vi "Periodic Tasks_Hue.vi"(8 "error in":errorcluster, 11 "RobotConfig":T7={"Motors"={"RightDrivePrimary"={"CAN Address"=0, "Invert"=FALSE, "InvertSensor"=FALSE, "Unit Conversion Factor"=0.0, "Brake Mode"=enum."Override to Brake", "Reverse Limt Switch Mode"=enum."Disabled", "Forward Limt Swith Mode"=enum."Disabled", "PWM Channel"=enum."Invalid", "Motor Controller Type"=enum."Talon SRX", "Peak Current (A)"=0, "Continuous Current (A)"=0, "Peak Duration (ms)"=0, "Current Limit Enable"=FALSE}, "RightDriveSecondary"={"CAN Address"=0, "Invert"=FALSE, "InvertSensor"=FALSE, "Unit Conversion Factor"=0.0, "Brake Mode"=enum."Override to Brake", "Reverse Limt Switch Mode"=enum."Disabled", "Forward Limt Swith Mode"=enum."Disabled", "PWM Channel"=enum."Invalid", "Motor Controller Type"=enum."Talon SRX", "Peak Current (A)"=0, "Continuous Current (A)"=0, "Peak Duration (ms)"=0, "Current Limit Enable"=FALSE}, "LeftDrivePrimary"={"CAN Address"=0, "Invert"=FALSE, "InvertSensor"=FALSE, "Unit Conversion Factor"=0.0, "Brake Mode"=enum."Override to Brake", "Reverse Limt Switch Mode"=enum."Disabled", "Forward Limt Swith Mode"=enum."Disabled", "PWM Channel"=enum."Invalid", "Motor Controller Type"=enum."Talon SRX", "Peak Current (A)"=0, "Continuous Current (A)"=0, "Peak Duration (ms)"=0, "Current Limit Enable"=FALSE}, "LeftDriveSecondary"={"CAN Address"=0, "Invert"=FALSE, "InvertSensor"=FALSE, "Unit Conversion Factor"=0.0, "Brake Mode"=enum."Override to Brake", "Reverse Limt Switch Mode"=enum."Disabled", "Forward Limt Swith Mode"=enum."Disabled", "PWM Channel"=enum."Invalid", "Motor Controller Type"=enum."Talon SRX", "Peak Current (A)"=0, "Continuous Current (A)"=0, "Peak Duration (ms)"=0, "Current Limit Enable"=FALSE}, "RightShooter"={"CAN Address"=0, "Invert"=FALSE, "InvertSensor"=FALSE, "Unit Conversion Factor"=0.0, "Brake Mode"=enum."Override to Brake", "Reverse Limt Switch Mode"=enum."Disabled", "Forward Limt Swith Mode"=enum."Disabled", "PWM Channel"=enum."Invalid", "Motor Controller Type"=enum."Talon SRX", "Peak Current (A)"=0, "Continuous Current (A)"=0, "Peak Duration (ms)"=0, "Current Limit Enable"=FALSE}, "LeftShooter"={"CAN Address"=0, "Invert"=FALSE, "InvertSensor"=FALSE, "Unit Conversion Factor"=0.0, "Brake Mode"=enum."Override to Brake", "Reverse Limt Switch Mode"=enum."Disabled", "Forward Limt Swith Mode"=enum."Disabled", "PWM Channel"=enum."Invalid", "Motor Controller Type"=enum."Talon SRX", "Peak Current (A)"=0, "Continuous Current (A)"=0, "Peak Duration (ms)"=0, "Current Limit Enable"=FALSE}, "ShooterRotate"={"CAN Address"=0, "Invert"=FALSE, "InvertSensor"=FALSE, "Unit Conversion Factor"=0.0, "Brake Mode"=enum."Override to Brake", "Reverse Limt Switch Mode"=enum."Disabled", "Forward Limt Swith Mode"=enum."Disabled", "PWM Channel"=enum."Invalid", "Motor Controller Type"=enum."Talon SRX", "Peak Current (A)"=0, "Continuous Current (A)"=0, "Peak Duration (ms)"=0, "Current Limit Enable"=FALSE}, "ShooterHood"={"CAN Address"=0, "Invert"=FALSE, "InvertSensor"=FALSE, "Unit Conversion Factor"=0.0, "Brake Mode"=enum."Override to Brake", "Reverse Limt Switch Mode"=enum."Disabled", "Forward Limt Swith Mode"=enum."Disabled", "PWM Channel"=enum."Invalid", "Motor Controller Type"=enum."Talon SRX", "Peak Current (A)"=0, "Continuous Current (A)"=0, "Peak Duration (ms)"=0, "Current Limit Enable"=FALSE}, "HopperWheel"={"CAN Address"=0, "Invert"=FALSE, "InvertSensor"=FALSE, "Unit Conversion Factor"=0.0, "Brake Mode"=enum."Override to Brake", "Reverse Limt Switch Mode"=enum."Disabled", "Forward Limt Swith Mode"=enum."Disabled", "PWM Channel"=enum."Invalid", "Motor Controller Type"=enum."Talon SRX", "Peak Current (A)"=0, "Continuous Current (A)"=0, "Peak Duration (ms)"=0, "Current Limit Enable"=FALSE}, "Elevator"={"CAN Address"=0, "Invert"=FALSE, "InvertSensor"=FALSE, "Unit Conversion Factor"=0.0, "Brake Mode"=enum."Override to Brake", "Reverse Limt Switch Mode"=enum."Disabled", "Forward Limt Swith Mode"=enum."Disabled", "PWM Channel"=enum."Invalid", "Motor Controller Type"=enum."Talon SRX", "Peak Current (A)"=0, "Continuous Current (A)"=0, "Peak Duration (ms)"=0, "Current Limit Enable"=FALSE}, "ClimberLeft"={"CAN Address"=0, "Invert"=FALSE, "InvertSensor"=FALSE, "Unit Conversion Factor"=0.0, "Brake Mode"=enum."Override to Brake", "Reverse Limt Switch Mode"=enum."Disabled", "Forward Limt Swith Mode"=enum."Disabled", "PWM Channel"=enum."Invalid", "Motor Controller Type"=enum."Talon SRX", "Peak Current (A)"=0, "Continuous Current (A)"=0, "Peak Duration (ms)"=0, "Current Limit Enable"=FALSE}, "ClimberRight"={"CAN Address"=0, "Invert"=FALSE, "InvertSensor"=FALSE, "Unit Conversion Factor"=0.0, "Brake Mode"=enum."Override to Brake", "Reverse Limt Switch Mode"=enum."Disabled", "Forward Limt Swith Mode"=enum."Disabled", "PWM Channel"=enum."Invalid", "Motor Controller Type"=enum."Talon SRX", "Peak Current (A)"=0, "Continuous Current (A)"=0, "Peak Duration (ms)"=0, "Current Limit Enable"=FALSE}, "Intake"={"CAN Address"=0, "Invert"=FALSE, "InvertSensor"=FALSE, "Unit Conversion Factor"=0.0, "Brake Mode"=enum."Override to Brake", "Reverse Limt Switch Mode"=enum."Disabled", "Forward Limt Swith Mode"=enum."Disabled", "PWM Channel"=enum."Invalid", "Motor Controller Type"=enum."Talon SRX", "Peak Current (A)"=0, "Continuous Current (A)"=0, "Peak Duration (ms)"=0, "Current Limit Enable"=FALSE}, "ControlPanel"={"CAN Address"=0, "Invert"=FALSE, "InvertSensor"=FALSE, "Unit Conversion Factor"=0.0, "Brake Mode"=enum."Override to Brake", "Reverse Limt Switch Mode"=enum."Disabled", "Forward Limt Swith Mode"=enum."Disabled", "PWM Channel"=enum."Invalid", "Motor Controller Type"=enum."Talon SRX", "Peak Current (A)"=0, "Continuous Current (A)"=0, "Peak Duration (ms)"=0, "Current Limit Enable"=FALSE}}, "PID"={"Shooter"={"P"=0.0, "I"=0.0, "D"=0.0, "F"=0.0, "IZone"=0.0}, "Turret"={"P"=0.0, "I"=0.0, "D"=0.0, "F"=0.0, "IZone"=0.0}, "Elevator"={"P"=0.0, "I"=0.0, "D"=0.0, "F"=0.0, "IZone"=0.0}, "ControlPanel"={"P"=0.0, "I"=0.0, "D"=0.0, "F"=0.0, "IZone"=0.0}, "Hood"={"P"=0.0, "I"=0.0, "D"=0.0, "F"=0.0, "IZone"=0.0}}, "MotionMagic"={"Turret"={"CruiseVelocity"=0, "Acceleration"=0}, "Elevator"={"CruiseVelocity"=0, "Acceleration"=0}, "ControlPanel"={"CruiseVelocity"=0, "Acceleration"=0}}, "Sensors"={"IMU"={"Yaw Axis"=enum."Z", "SPI Bus"=enum."SPI MXP", "AHRS Algorithm"=enum."Complementary", "Calibration Time (s)"=3.0, "Calibrate On Open"=TRUE}, "ElevatorBottom"={"ID"=0, "RangingMode"=enum."Short", "sampleTime(ms)"=24.0}, "ElevatorTop"={"ID"=0, "RangingMode"=enum."Short", "sampleTime(ms)"=24.0}}, "Solenoids"={"Intake"={"SolenoidChannel"=enum."Solenoid 0", "Invert"=FALSE}, "ClimberRachet"={"SolenoidChannel"=enum."Solenoid 0", "Invert"=FALSE}}, "EnableCompressor"=FALSE, "RobotDimensions"={"Wheelbase(in)"=0.0, "Length(in)"=0.0}, "CameraMounting"={"LensHeight(in)"=0.0, "RotationRadius(in)"=0.0, "Pitch(deg)"=0.0}, "SensorCalibrations"={"TopToFMinBallDistance(in)"=0.0, "BottomToFMinBallDistance(in)"=0.0}, "Homing"={"Hood Homing Position (deg)"=0.0, "Turret Homing Position (deg)"=0.0}, "MotionLimits"={"Hood"={"Min (deg)"=0.0, "Max (deg)"=0.0}, "Turret"={"Min (deg)"=0.0, "Max (deg)"=0.0}}} {"Sensors"."ElevatorTop"."sampleTime(ms)" min=24.0 max=1000.0 step=1.0; "Sensors"."ElevatorBottom"."sampleTime(ms)" min=24.0 max=1000.0 step=1.0}) -> ()   [LabVIEW 2019]
doc: "This VI runs in parallel to other tasks. It can contain as many user-defined periodic loops as you need. These can carry out PID or other sorts of timed response."
uses:
  InfiniteRechargeSrc/TypeDefs/ConfigComponents/Config_Robot.ctl
  ArgosLib/Config/ConfigComponents/TypeDefs/Config_Motor.ctl
  <vilib>/Rock Robotics/WPI/ThirdParty/Phoenix-LabVIEW/Motor Controller/Controls/CTRE_Phoenix_MotorControl_NeutralMode.ctl
  <vilib>/Rock Robotics/WPI/ThirdParty/Phoenix-LabVIEW/Motor Controller/Controls/CTRE_Phoenix_MotorControl_LimitSwitchNormal.ctl
  <vilib>/Rock Robotics/SystemInterfaces/DIO/FPGA_DIOPWMChannel.ctl
  ArgosLib/Config/ConfigComponents/TypeDefs/Config_MotorCtrlType.ctl
  ArgosLib/Config/ConfigComponents/TypeDefs/Config_PIDParams.ctl
  ArgosLib/Config/ConfigComponents/TypeDefs/Config_MotionMagicParams.ctl
  ArgosLib/Config/ConfigComponents/TypeDefs/Config_IMU.ctl
  <vilib>/Rock Robotics/SystemInterfaces/spilib/spi_bus.ctl
  ArgosLib/Config/ConfigComponents/TypeDefs/Config_PwFToF.ctl
  <vilib>/Playing With Fusion Inc/Playing With Fusion Lib for FRC/PWF_ToF_LabVIEW/Public/TypeDefs/PwF_ToF_RangingMode.ctl
  ArgosLib/Config/ConfigComponents/TypeDefs/Config_SingleSolenoid.ctl
  <vilib>/Rock Robotics/WPI/Solenoid/WPI_SolenoidChannel.ctl
  InfiniteRechargeSrc/TypeDefs/ConfigComponents/Config_RobotDimensions.ctl
  InfiniteRechargeSrc/TypeDefs/ConfigComponents/Config_CameraMounting.ctl
  ArgosLib/Miscellaneous/TypeDefs/ArgoDriveJoystickMap.ctl
  ArgosLib/Miscellaneous/TypeDefs/LookUpTableParameters.ctl
  InfiniteRechargeSrc/Implements/Shooter/TypeDefs/Hood_Homing_State.ctl
  <vilib>/Playing With Fusion Inc/Playing With Fusion Lib for FRC/PWF_TMD37003_LabVIEW/Public/TypeDefs/PwF_TMD37003_Data.ctl
  <vilib>/Playing With Fusion Inc/Playing With Fusion Lib for FRC/PWF_TMD37003_LabVIEW/Public/TypeDefs/PwF_TMD37003_Gains.ctl
  InfiniteRechargeSrc/Implements/Control_Panel/TypeDefs/ControlPanelColor.ctl
  InfiniteRechargeSrc/Vision/TypeDefs/VisionPipeline.ctl
  <vilib>/Rock Robotics/WPI/Utilities/WPI_GetSetVariantRefNum.vi
  InfiniteRechargeSrc/Global_Var-RefNum/JoystickControls.vi
  <vilib>/Playing With Fusion Inc/Playing With Fusion Lib for FRC/PWF_TMD37003_LabVIEW/Public/PwF_TMD37003_RGBToHSV_SensorData.vi
  ArgosLib/ArgosLib.lvlib
  <vilib>/Playing With Fusion Inc/Playing With Fusion Lib for FRC/PWF_TMD37003_LabVIEW/PwF_TMD37003.lvlib
  <vilib>/Playing With Fusion Inc/Playing With Fusion Lib for FRC/PWF_ToF_LabVIEW/PwF_ToF.lvlib
panel:
  out "Color":T1
  out "Hue":dbl
  in  "TMD37003Gains":T2={"rGain"=5.0761, "gGain"=7.9365, "bGain"=14.0845, "cGain"=2.9411, "gamma"=0.4545}
  in  "alsGain":u8=40
  in  "alsIntegrationTime(ms)":dbl=10.0
  out "TMD37003 Data":T3
  in  "ShooterSpeed(rpm)":dbl(slide)=4000.0 min=0.0 max=7000.0 step=1.0 scale=0.0..7000.0
  in  "DisableLimelight":bool
  out "Target Found?":bool
  in  "SetPointTurret(Deg)":dbl(slide) scale=-108.0..108.0
  in  "Activate Auto (Turret)":bool
  out "TurretManual":bool
  out "Turret Current Position (Deg)":dbl
  out "Hood Current Position (Deg)":dbl
  out "HoodManual?":bool
  in  "Activate Auto (Shooter Hood)":bool
  in  "SetPointHood(Deg)":dbl
  in  "TurretHomeReset":bool
  in  "Turret Homing Activated":bool
  out "Turret Homing_State":T4
  in  "HoodHomeActivate":bool
  in  "HoodHomeReset":bool
  out "Hood_Homing_State":T4
  in  "Argo Drive Joystick Map":T5={"Auto Speed"={"Look Up Table OUT"=[-1.0, 0.0, 1.0], "Look Up Table IN"=[-1.0, 0.0, 1.0]}, "Low Speed"={"Look Up Table OUT"=[-1.0, 0.0, 0.0, 1.0], "Look Up Table IN"=[-1.0, -0.25, 0.25, 1.0]}, "Auto Turning"={"Look Up Table OUT"=[-1.0, 0.0, 1.0], "Look Up Table IN"=[-1.0, 0.0, 1.0]}, "Low Turning"={"Look Up Table OUT"=[-1.0, 0.0, 0.0, 1.0], "Look Up Table IN"=[-1.0, -0.25, 0.25, 1.0]}, "High Speed"={"Look Up Table OUT"=[], "Look Up Table IN"=[]}, "High Turning"={"Look Up Table OUT"=[], "Look Up Table IN"=[]}}
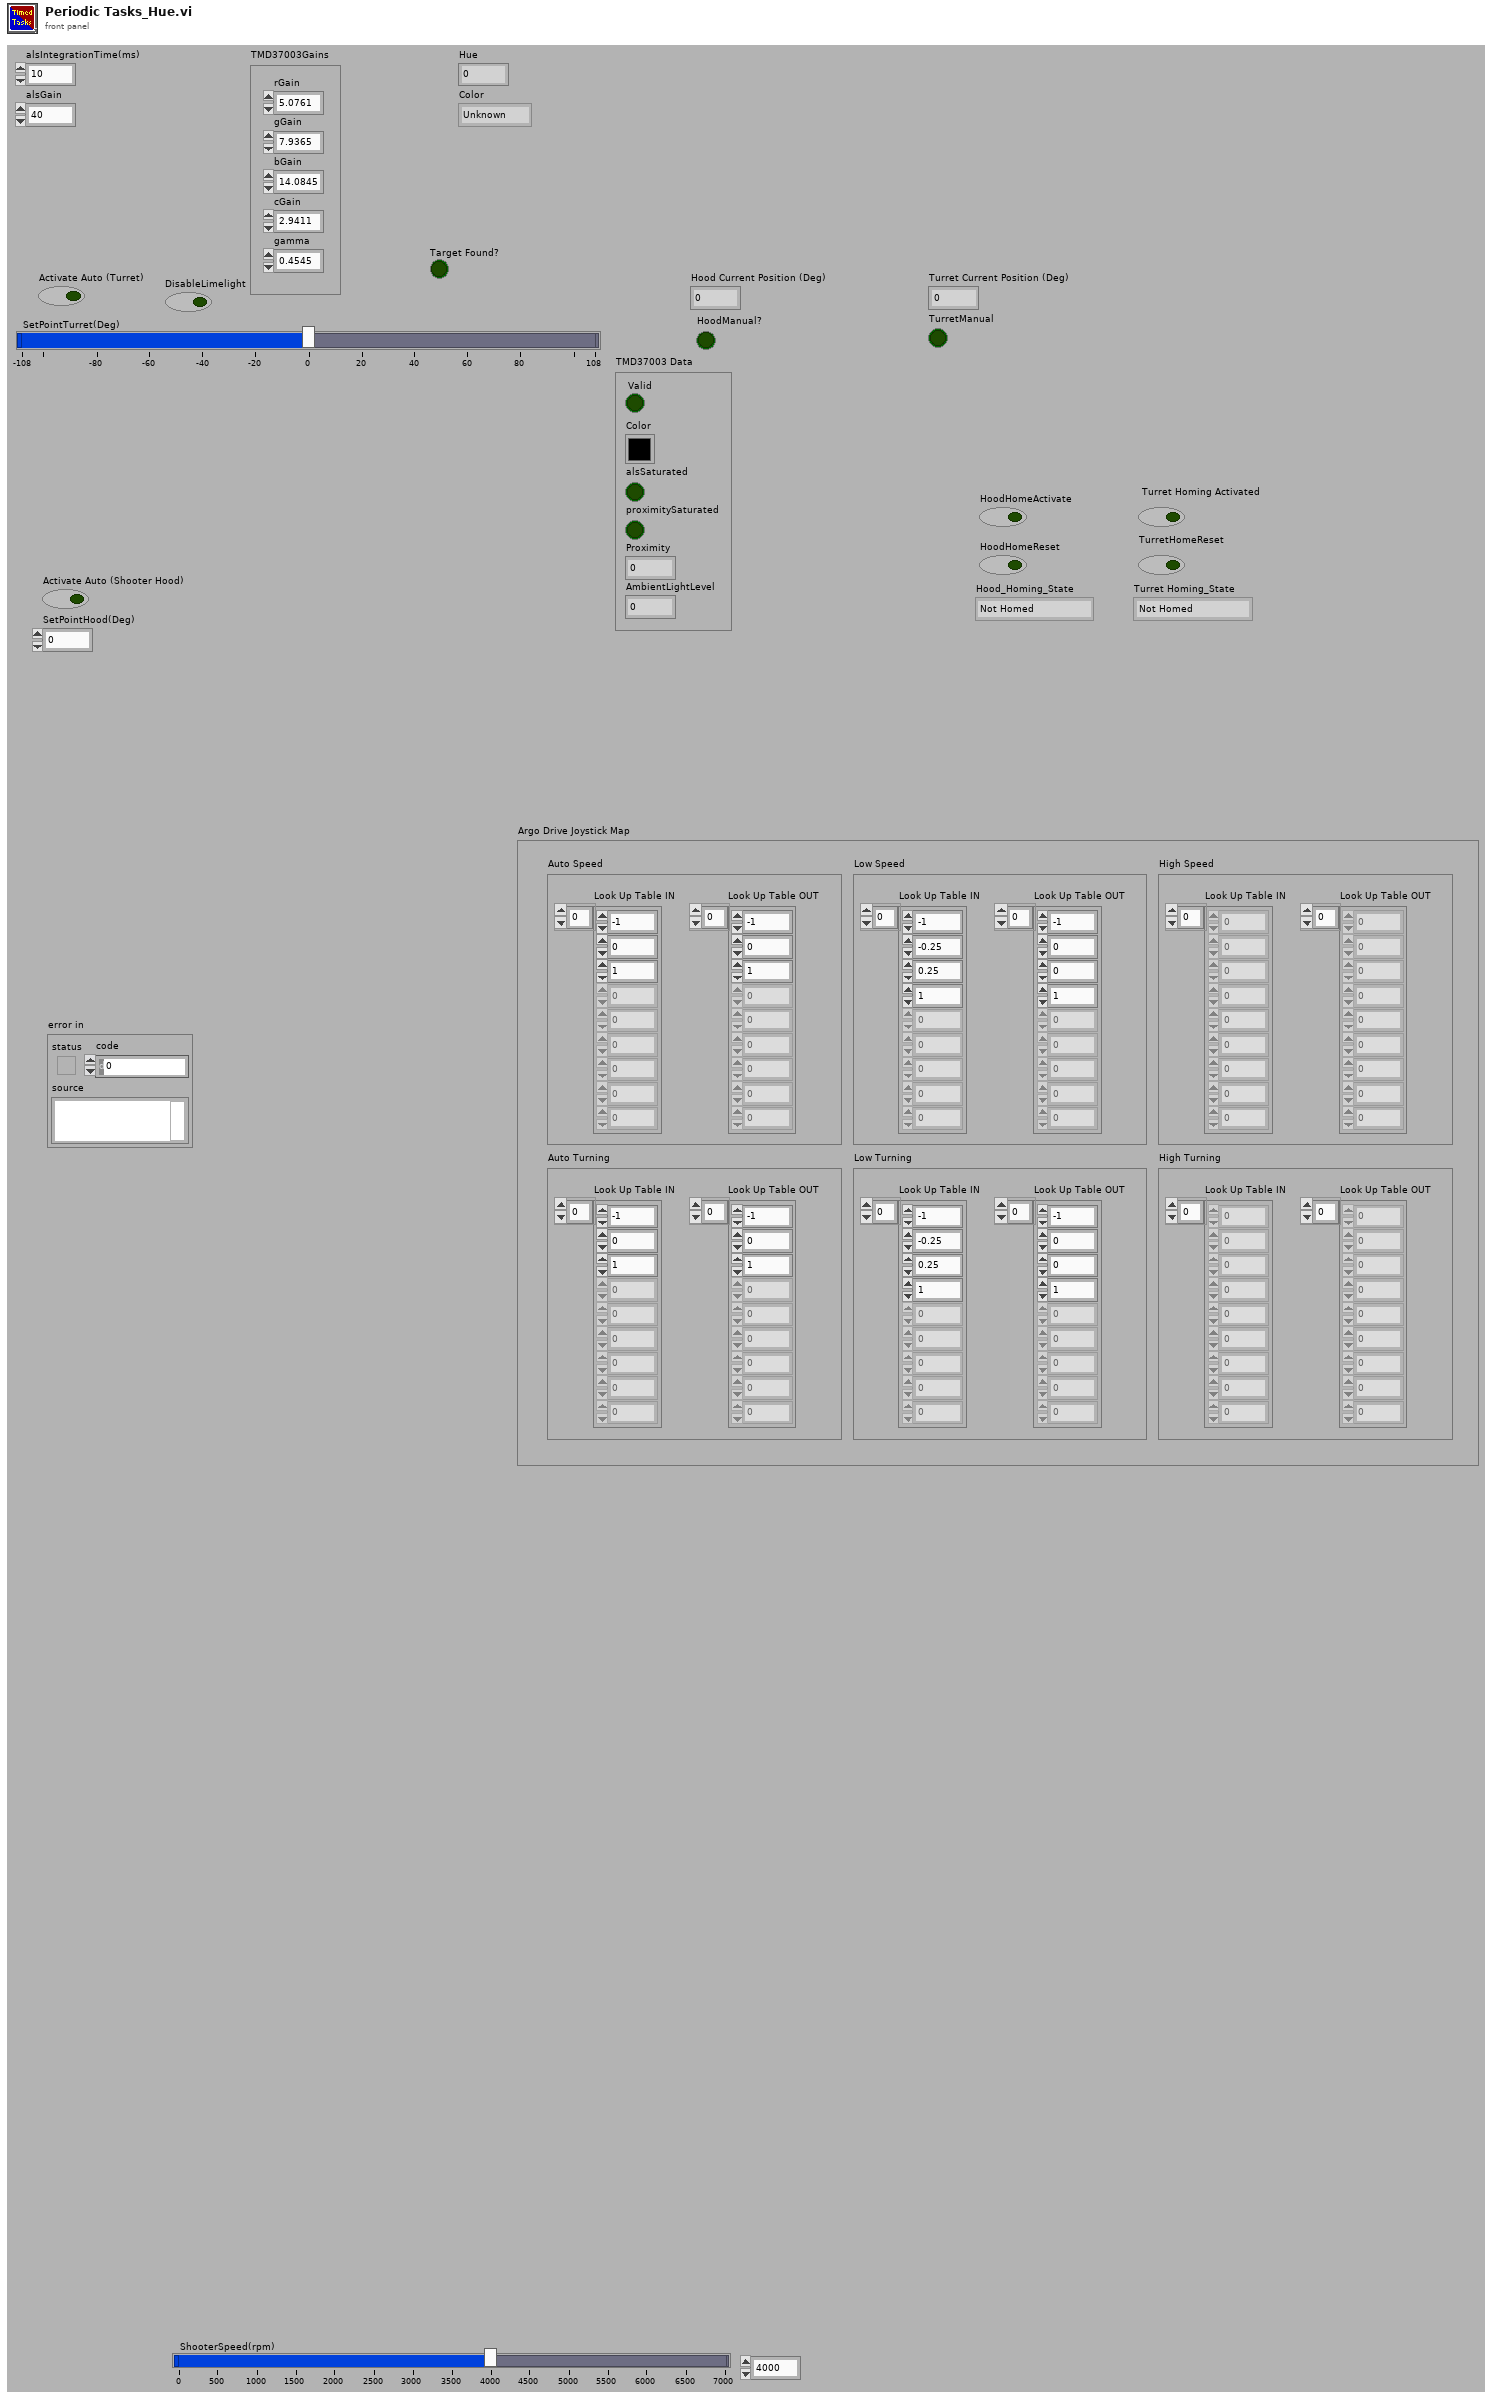
[diagram p1: front panel]
types:
  T1 = typedef "ControlPanelColor.ctl" = enum16{"Unknown", "Red", "Green", "Blue", "Yellow"}
  T2 = typedef "PlayingWithFusionLib.lvlib/PwF_TMD37003.lvlib/PwF_TMD37003_Gains.ctl" = cluster{"rGain":dbl, "gGain":dbl, "bGain":dbl, "cGain":dbl, "gamma":dbl}
  T3 = typedef "PlayingWithFusionLib.lvlib/PwF_TMD37003.lvlib/PwF_TMD37003_Data.ctl" = cluster{"Valid":bool, "Color":u32, "alsSaturated":bool, "proximitySaturated":bool, "Proximity":dbl, "AmbientLightLevel":dbl}
  T4 = typedef "Hood_Homing_State.ctl" = enum16{"Not Homed", "Homing in Process", "Homing Failed", "Homing Completed"}
  T5 = typedef "ArgosLib.lvlib/ArgoDriveJoystickMap.ctl" = cluster{"Auto Speed":T6, "Low Speed":T6, "Auto Turning":T6, "Low Turning":T6, "High Speed":T6, "High Turning":T6}
  T6 = typedef "ArgosLib.lvlib/LookUpTableParameters.ctl" = cluster{"Look Up Table OUT":dbl[], "Look Up Table IN":dbl[]}
  T7 = typedef "Config_Robot.ctl" = cluster{"Motors":cluster{"RightDrivePrimary":T8, "RightDriveSecondary":T8, "LeftDrivePrimary":T8, "LeftDriveSecondary":T8, "RightShooter":T8, "LeftShooter":T8, "ShooterRotate":T8, "ShooterHood":T8, "HopperWheel":T8, "Elevator":T8, "ClimberLeft":T8, "ClimberRight":T8, "Intake":T8, "ControlPanel":T8}, "PID":cluster{"Shooter":T13, "Turret":T13, "Elevator":T13, "ControlPanel":T13, "Hood":T13}, "MotionMagic":cluster{"Turret":T14, "Elevator":T14, "ControlPanel":T14}, "Sensors":cluster{"IMU":T15, "ElevatorBottom":T17, "ElevatorTop":T17}, "Solenoids":cluster{"Intake":T19, "ClimberRachet":T19}, "EnableCompressor":bool, "RobotDimensions":T21, "CameraMounting":T22, "SensorCalibrations":cluster{"TopToFMinBallDistance(in)":dbl, "BottomToFMinBallDistance(in)":dbl}, "Homing":cluster{"Hood Homing Position (deg)":dbl, "Turret Homing Position (deg)":dbl}, "MotionLimits":cluster{"Hood":cluster{"Min (deg)":dbl, "Max (deg)":dbl}, "Turret":cluster{"Min (deg)":dbl, "Max (deg)":dbl}}}
  T8 = typedef "ArgosLib.lvlib/Config_Motor.ctl" = cluster{"CAN Address":u8, "Invert":bool, "InvertSensor":bool, "Unit Conversion Factor":dbl, "Brake Mode":T9, "Reverse Limt Switch Mode":T10, "Forward Limt Swith Mode":T10, "PWM Channel":T11, "Motor Controller Type":T12, "Peak Current (A)":i32, "Continuous Current (A)":i32, "Peak Duration (ms)":i32, "Current Limit Enable":bool}
  T9 = typedef "CTRE_Phoenix_MotorControl_NeutralMode.ctl" = enum8{"EEPROMSetting", "Override to Coast", "Override to Brake"}
  T10 = typedef "CTRE_Phoenix_MotorControl_LimitSwitchNormal.ctl" = enum16{"Normally Open", "Normally Closed", "Disabled"}
  T11 = typedef "FPGA_DIOPWMChannel.ctl" = enum8{"PWM 0", "PWM 1", "PWM 2", "PWM 3", "PWM 4", "PWM 5", "PWM 6", "PWM 7", "PWM 8", "PWM 9", "PWM MXP 0", "PWM MXP 1", "PWM MXP 2", "PWM MXP 3", "PWM MXP 4", "PWM MXP 5", "PWM MXP 6", "PWM MXP 7", "PWM MXP 8", "PWM MXP 9", "Invalid"}
  T12 = typedef "ArgosLib.lvlib/Config_MotorCtrlType.ctl" = enum16{"Disabled", "Talon SRX", "Talon SR", "Venom", "Spark MAX"}
  T13 = typedef "ArgosLib.lvlib/Config_PIDParams.ctl" = cluster{"P":dbl, "I":dbl, "D":dbl, "F":dbl, "IZone":dbl}
  T14 = typedef "ArgosLib.lvlib/Config_MotionMagicParams.ctl" = cluster{"CruiseVelocity":i32, "Acceleration":i32}
  T15 = typedef "ArgosLib.lvlib/Config_IMU.ctl" = cluster{"Yaw Axis":enum16{"X", "Y", "Z"}, "SPI Bus":T16, "AHRS Algorithm":enum16{"Complementary", "Madgwick"}, "Calibration Time (s)":dbl, "Calibrate On Open":bool}
  T16 = typedef "spi_bus.ctl" = enum16{"SPI On-Board, CS0", "SPI On-Board, CS1", "SPI On-Board, CS2", "SPI On-Board, CS3", "SPI MXP", "Invalid"}
  T17 = typedef "ArgosLib.lvlib/Config_PwFToF.ctl" = cluster{"ID":u8, "RangingMode":T18, "sampleTime(ms)":dbl}
  T18 = typedef "PlayingWithFusionLib.lvlib/PwF_ToF.lvlib/PwF_ToF_RangingMode.ctl" = enum16{"Short", "Medium", "Long"}
  T19 = typedef "ArgosLib.lvlib/Config_SingleSolenoid.ctl" = cluster{"SolenoidChannel":T20, "Invert":bool}
  T20 = typedef "WPI_SolenoidChannel.ctl" = enum8{"Solenoid 0", "Solenoid 1", "Solenoid 2", "Solenoid 3", "Solenoid 4", "Solenoid 5", "Solenoid 6", "Solenoid 7", "Invalid"}
  T21 = typedef "Config_RobotDimensions.ctl" = cluster{"Wheelbase(in)":dbl, "Length(in)":dbl}
  T22 = typedef "Config_CameraMounting.ctl" = cluster{"LensHeight(in)":dbl, "RotationRadius(in)":dbl, "Pitch(deg)":dbl}
  T23 = typedef "SensorRefNums.ctl" = cluster{"ElevatorBottom":T24, "ElevatorTop":T24}
  T24 = typedef "PlayingWithFusionLib.lvlib/PwF_ToF.lvlib/PwF_ToF_DevRef.ctl" = cluster{"DeviceStatus":errorcluster, "Device Number":u8, "Handle":u64, "Library Path":path}
  T25 = typedef "JoystickRefNums.ctl" = cluster{"Joystick0":T26, "Joystick1":T26}
  T26 = typedef "WPI_JoystickDevRef.ctl" = cluster{"Device":T27}
  T27 = typedef "WPI_JoystickDeviceEnum.ctl" = enum16{"USB 0", "USB 1", "USB 2", "USB 3", "USB 4", "USB 5"}
  T28 = typedef "WPI_RobotDriveDevRef.ctl" = cluster{"DevStatus":errorcluster, "Motors[]":T29[], "Square Inputs":bool, "Max Output":dbl}
  T29 = typedef "WPI_MotorControlDeviceRef.ctl" = cluster{"DeviceStatus":errorcluster, "Type":T30, "PWM":cluster{"PWM Channel":T11, "DeadBand":T31}, "CAN":cluster{"Device Number":u8, "SetOutput VI Ref":variant, "GetOutput VI Ref":variant, "Enable VI Ref":variant, "Disable VI Ref":variant, "Data":variant}, "Invert":bool, "DIO PWM":cluster{"PWM \"Enable\" Channel":T11, "DIOChannel":T32, "PWM Rate":dbl}}
  T30 = typedef "WPI_MotorControlType.ctl" = enum16{"PWM", "CAN", "DIO PWM"}
  T31 = typedef "WPI_PWMDeadband.ctl" = cluster{"Name":string, "maxPositivePwm":i32, "minPositivePwm":i32, "centerPwm":i32, "maxNegativePwm":i32, "minNegativePwm":i32, "angularRange":u16}
  T32 = typedef "FPGA_DIOChannel.ctl" = enum8{"DIO 0", "DIO 1", "DIO 2", "DIO 3", "DIO 4", "DIO 5", "DIO 6", "DIO 7", "DIO 8", "DIO 9", "DIO MXP 0", "DIO MXP 1", "DIO MXP 2", "DIO MXP 3", "DIO MXP 4", "DIO MXP 5", "DIO MXP 6", "DIO MXP 7", "DIO MXP 8", "DIO MXP 9", "DIO MXP 10", "DIO MXP 11", "DIO MXP 12", "DIO MXP 13", "DIO MXP 14", "DIO MXP 15", "SPI Port CS1", "SPI Port CS2", "SPI Port CS3", "SPI Port MISO", "SPI Port MOSI", "Invalid"}
  T33 = typedef "PneumaticsRefNums.ctl" = cluster{"Intake":T34, "Compressor":T35, "ClimberRatchet":T34}
  T34 = typedef "WPI_SolenoidDevRef.ctl" = cluster{"DevStatus":errorcluster, "Pneumatics Control Module":u8, "Forward Solenoid Channel":T20, "Reverse Solenoid Channel":T20}
  T35 = typedef "WPI_CompressorDevRef.ctl" = cluster{"DevStatus":errorcluster, "Pneumatics Control Module":u8}
  T36 = typedef "MotorRefNums.ctl" = cluster{"LeftDrivePrimary":T29, "RightDrivePrimary":T29, "LeftDriveSecondary":T29, "RightDriveSecondary":T29, "RightShooter":T29, "LeftShooter":T29, "ShooterRotate":T29, "ShooterHood":T29, "HopperWheel":T29, "Elevator":T29, "ClimberLeft":T29, "ClimberRight":T29, "Intake":T29, "ControlPanel":T29}
  T37 = cluster{"RobotConfig":T7, "JoystickRefNums":T25, "RobotDriveDevRef":T28, "MotorRefNumsOut":T36, "Pneumatics":T33, "Sensors":T23}
  T38 = typedef "PlayingWithFusionLib.lvlib/PwF_TMD37003.lvlib/PwF_TMD37003_DevRef.ctl" = cluster{"DevStatus":errorcluster, "Device Address":u8, "Handle":i32, "I2C Bus":T39}
  T39 = typedef "i2c_bus.ctl" = enum16{"I2C On-Board", "I2C MXP", "Invalid"}
  T40 = typedef "JoystickControl.ctl" = cluster{"A":bool, "B":bool, "X":bool, "Y":bool, "LB":bool, "Shoot":bool, "LJ":bool, "RJ":bool, "Back":bool, "Start":bool, "Top":bool, "Right":bool, "Bottom":bool, "Left":bool, "Eject":dbl, "Intake":dbl, "LX":dbl, "Drive Y":dbl, "Drive X":dbl, "RY":dbl, "Down":bool, "Index":bool, "Aggitate":bool, "Up":bool, "Find Target":bool, "Spin up":bool, "LJ 2":bool, "RJ 2":bool, "Back 2":bool, "Start 2":bool, "Elevate":bool, "Right 2":bool, "Retract":bool, "Left 2":bool, "Control Rotate":dbl, "RT 2":dbl, "H L/R":dbl, "H U/D":dbl, "RX 2":dbl, "RY 2":dbl}
  T41 = typedef "VisionPipeline.ctl" = enum16{"LEDOff", "NoZoom", "Zoom2x", "Zoom3x"}
  T42 = typedef "VisionTarget.ctl" = cluster{"Valid":bool, "Distance(in)":dbl, "Angle(deg)":dbl, "FieldCentricAngle(deg)":dbl}
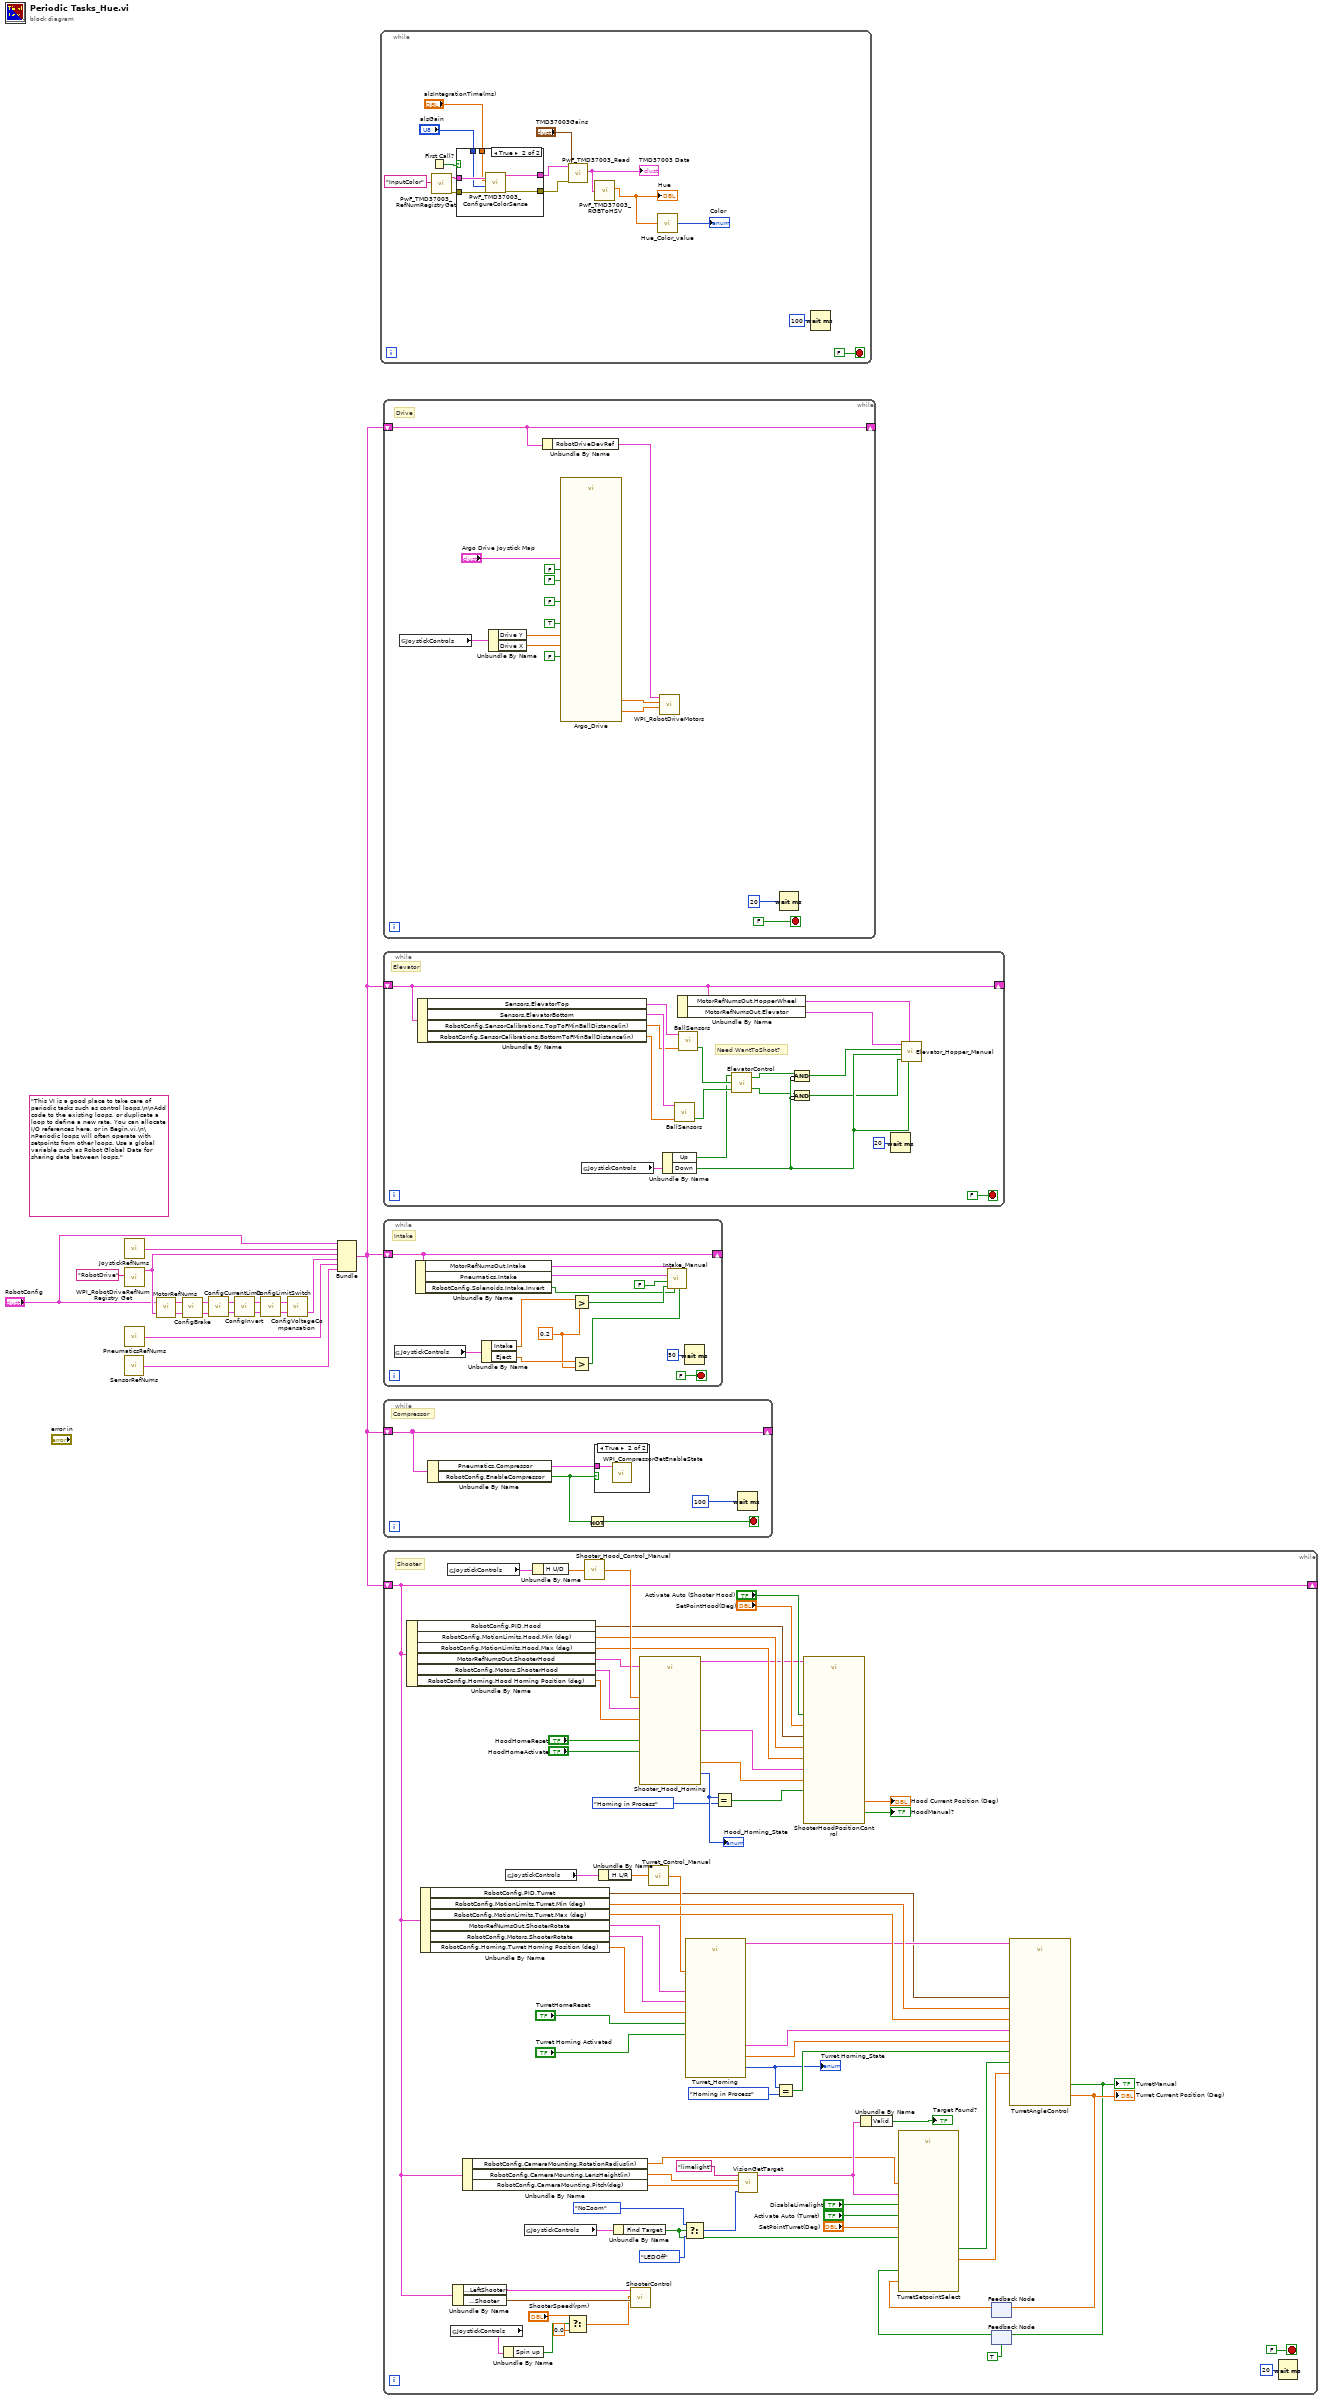
[diagram p0: block diagram]
diagram:
  (unwired) "This VI is a good place to take care of periodic tasks such as control loops.\n\nAdd code to the existing loops, or duplicate a loop to define a new rate. You can allocate I/O references here, or in Begin.vi.\n\nPeriodic loops will often operate with setpoints from other loops. Use a global variable such as Robot Global Data for sharing data between loops."
  n1 = call "SensorRefNums.vi"() -> ("Sensors"=w14:T23)  [unwired: 1 in]
  n2 = call "JoystickRefNums.vi"() -> ("JoystickRefNums"=w18:T25)  [unwired: 1 in]
  n3 = call <vilib>:"WPI_RobotDriveRefNum Registry Get.vi"("refnum name"="RobotDrive") -> ("RobotDriveDevRef"=w16:T28)  [unwired: 9 in, 1 out]
  n4 = call "PneumaticsRefNums.vi"() -> ("Pneumatics"=w15:T33)  [unwired: 1 in]
  n5 = call "MotorRefNums.vi"("RobotDriveDevRef"=w16, "RobotConfig"="RobotConfig") -> ("MotorRefNums"=w12:T36, "RobotConfigOut"=w13:T7)
  n6 = call "ConfigBrake.vi"("MotorRefNumsIn"=w12, "RobotConfigIn"=w13) -> ("MotorRefNumsOut"=w11:T36, "RobotConfigOut"=w10:T7)
  n7 = call "ConfigCurrentLimit.vi"("MotorRefNumsIn"=w11, "RobotConfigIn"=w10) -> ("MotorRefNumsOut"=w9:T36, "RobotConfigOut"=w8:T7)
  n8 = call "ConfigInvert.vi"("MotorRefNumsIn"=w9, "RobotConfigIn"=w8) -> ("MotorRefNumsOut"=w7:T36, "RobotConfigOut"=w6:T7)
  n9 = call "ConfigLimitSwitch.vi"("MotorRefNumsIn"=w7, "RobotConfigIn"=w6) -> ("MotorRefNumsOut"=w5:T36, "RobotConfigOut"=w4:T7)
  n10 = call "ConfigVoltageCompensation.vi"("MotorRefNumsIn"=w5, "RobotConfigIn"=w4) -> ("MotorRefNumsOut"=w3:T36)  [unwired: 1 out]
  n11 = Bundle("RobotConfig"="RobotConfig", "JoystickRefNums"=w18, "RobotDriveDevRef"=w16, "MotorRefNumsOut"=w3, "Pneumatics"=w15, "Sensors"=w14) -> (w1:T37)  [unwired: 1 out]
  n12 = while {
    stop <- FALSE stop-if-true
    n13 = First Call?() -> (First Call?: T/F=w29:bool)
    n14 = call <vilib>:"PwF_TMD37003_RefNumRegistryGet.vi"("refnum name"="InputColor") -> ("error out"=w27:errorcluster, "PwFTMD37003DevRefOut"=w28:T38)  [unwired: 9 in]
    n15 = case shown="True" w29 {
      tunnel: w28 -> [w34 w40]
      tunnel: [w34 w39] -> w23
      tunnel: w27 -> [w33 w38]
      tunnel: [w33 w37] -> w22
      tunnel: "alsIntegrationTime(ms)" -> [_ w36]
      tunnel: "alsGain" -> [_ w35]
      frame False {
      }
      frame True {
        n16 = call <vilib>:"PwF_TMD37003_ConfigureColorSense.vi"("error in (no error)"=w38, "alsGain"=w35, "alsIntegrationTime(ms)"=w36, "PwF_TMD37003_DevRefIn"=w40) -> ("error out"=w37:errorcluster, "PwF_TMD37003_DevRefOut"=w39:T38)  [unwired: 6 in]
      }
    }
    n17 = call <vilib>:"PwF_TMD37003_Read.vi"("error in (no error)"=w22, "TMD37003Gains"="TMD37003Gains", "PwF_TMD37003_DevRefIn"=w23) -> ("TMD37003 Data"=w20:T3)  [unwired: 6 in, 2 out]
    "TMD37003 Data" <- w20
    n18 = call-poly <vilib>:"PwF_TMD37003_RGBToHSV.vi"("TMD37003 Data In"=w20) -> ("Hue"=w19:dbl)  [unwired: 3 out]
    "Hue" <- w19
    n19 = call "Hue_Color_value.vi"("Hue"=w19) -> ("Color"=→"Color":T1)
    n20 = Wait (ms)(milliseconds to wait=u32 100) -> ()  [unwired: 1 out]
  }
  n21 = while {
    shift-right: [w53] -> _
    shift-left: w1 -> [w53]
    stop <- FALSE stop-if-true
    # "Drive"
    n22 = global read "JoystickControls.vi" "JoystickControls"() -> (w52:T40)
    n23 = Unbundle By Name(w52) -> ("Drive Y"=w51:dbl, "Drive X"=w50:dbl)
    n24 = Unbundle By Name(w53) -> ("RobotDriveDevRef"=w43:T28)
    n25 = call "Argo_Drive.vi"("Speed_Main"=w51, "Argo Drive Joystick Map"="Argo Drive Joystick Map", "Backwards_Turning_Flip"=FALSE, "Turning_PID_Enable"=FALSE, "Turning_Main"=w50, "Auto_Enable"=FALSE, "High_Gear"=FALSE, "Quick_Turn"=TRUE) -> ("Left_Motor"=w42:dbl, "Right_Motor"=w41:dbl)  [unwired: 10 in]
    n26 = call <vilib>:"WPI_RobotDriveMotors.vi"("RightSpeed"=w41, "LeftSpeed"=w42, "RobotDriveDevRef"=w43) -> ()  [unwired: 6 in, 3 out]
    n27 = Wait (ms)(milliseconds to wait=u32 20) -> ()  [unwired: 1 out]
  }
  n28 = while {
    shift-right: [w67] -> _
    shift-left: w1 -> [w67]
    stop <- FALSE stop-if-true
    # "Need WantToShoot?"
    # "Elevator"
    n29 = Unbundle By Name(w67) -> ("Sensors.ElevatorTop"=w69:T24, "Sensors.ElevatorBottom"=w68:T24, "RobotConfig.SensorCalibrations.TopToFMinBallDistance(in)"=w59:dbl, "RobotConfig.SensorCalibrations.BottomToFMinBallDistance(in)"=w58:dbl)
    n30 = global read "JoystickControls.vi" "JoystickControls"() -> (w66:T40)
    n31 = Unbundle By Name(w66) -> ("Up"=w60:bool, "Down"=w65:bool)
    n32 = call "BallSensors.vi"("MinDistance(in.)"=w58, "BallSensorDevRefIn"=w68) -> ("BallThere?"=w71:bool)  [unwired: 1 in, 2 out]
    n33 = Unbundle By Name(w67) -> ("MotorRefNumsOut.HopperWheel"=w56:T29, "MotorRefNumsOut.Elevator"=w57:T29)
    n34 = call "BallSensors.vi"("MinDistance(in.)"=w59, "BallSensorDevRefIn"=w69) -> ("BallThere?"=w70:bool)  [unwired: 1 in, 2 out]
    n35 = call "ElevatorControl.vi"("BallThereAtBottom?"=w71, "BallThereAtTop?"=w70, "WantToShoot?"=w60) -> ("HopperWheelsOn"=w63:bool, "ElevatorOn"=w64:bool)
    n36 = Compound Arithmetic op=AND(w64, invert w65) -> (w62:bool)
    n37 = Compound Arithmetic op=AND(w63, invert w65) -> (w61:bool)
    n38 = Wait (ms)(milliseconds to wait=u32 20) -> ()  [unwired: 1 out]
    n39 = call "Elevator_Hopper_Manual.vi"("Elevator_Control"=w57, "Hopper_Control"=w56, "Elevator_up"=w62, "Elevator_Down"=w65, "Hopper Backwards"=w65, "Hopper Forwards"=w61) -> ()  [unwired: 3 in]
  }
  n40 = while {
    shift-right: [w80] -> _
    shift-left: w1 -> [w80]
    stop <- FALSE stop-if-true
    w75 = 0.2 ("y")
    # "Intake"
    n41 = global read "JoystickControls.vi" "JoystickControls"() -> (w84:T40)
    n42 = Unbundle By Name(w80) -> ("MotorRefNumsOut.Intake"=w79:T29, "Pneumatics.Intake"=w78:T34, "RobotConfig.Solenoids.Intake.Invert"=w74:bool)
    n43 = Unbundle By Name(w84) -> ("Intake"=w77:dbl, "Eject"=w76:dbl)
    n44 = Greater?(x=w77, y=w75) -> (0:w81:bool)
    n45 = Greater?(x=w76, y=w75) -> (0:w82:bool)
    n46 = call "Intake_Manual.vi"("Reverse_Intake"=w82, "Invert Solenoid"=w74, "Intake"=w81, "Disable"=FALSE, "IntakeExtendDevRef"=w78, "Intake_Motor"=w79) -> ()  [unwired: 5 in]
    n47 = Wait (ms)(milliseconds to wait=u32 50) -> ()  [unwired: 1 out]
  }
  n48 = while {
    shift-right: [w90] -> _
    shift-left: w1 -> [w90]
    stop <- w88 stop-if-true
    # "Compressor"
    n49 = Unbundle By Name(w90) -> ("Pneumatics.Compressor"=w89:T35, "RobotConfig.EnableCompressor"=w87:bool)
    n50 = Not(x=w87) -> (.not. x?=w88:bool)
    n51 = case shown="True" w87 {
      tunnel: w89 -> [_ w92]
      frame False {
      }
      frame True {
        n52 = call <vilib>:"WPI_CompressorGetEnableState.vi"("CompressorDevRef"=w92) -> ()  [unwired: 7 in, 4 out]
      }
    }
    n53 = Wait (ms)(milliseconds to wait=u32 100) -> ()  [unwired: 1 out]
  }
  n54 = while {
    shift-right: [w93] -> _
    shift-left: w1 -> [w93]
    stop <- FALSE stop-if-true
    # "Shooter"
    n55 = Unbundle By Name(w93) -> ("RobotConfig.PID.Hood"=w119:T13, "RobotConfig.MotionLimits.Hood.Min (deg)"=w142:dbl, "RobotConfig.MotionLimits.Hood.Max (deg)"=w143:dbl, "MotorRefNumsOut.ShooterHood"=w152:T29, "RobotConfig.Motors.ShooterHood"=w153:T8, "RobotConfig.Homing.Hood Homing Position (deg)"=w154:dbl)
    n56 = Unbundle By Name(w93) -> ("RobotConfig.PID.Turret"=w101:T13, "RobotConfig.MotionLimits.Turret.Min (deg)"=w137:dbl, "RobotConfig.MotionLimits.Turret.Max (deg)"=w138:dbl, "MotorRefNumsOut.ShooterRotate"=w105:T29, "RobotConfig.Motors.ShooterRotate"=w103:T8, "RobotConfig.Homing.Turret Homing Position (deg)"=w136:dbl)
    n57 = global read "JoystickControls.vi" "JoystickControls"() -> (w157:T40)
    n58 = global read "JoystickControls.vi" "JoystickControls"() -> (w98:T40)
    n59 = Unbundle By Name(w93) -> ("MotorRefNumsOut.LeftShooter"=w100:T29, "RobotConfig.PID.Shooter"=w99:T13)
    n60 = Unbundle By Name(w93) -> ("RobotConfig.CameraMounting.RotationRadius(in)"=w106:dbl, "RobotConfig.CameraMounting.LensHeight(in)"=w128:dbl, "RobotConfig.CameraMounting.Pitch(deg)"=w127:dbl)
    n61 = Unbundle By Name(w98) -> ("Spin up"=w97:bool)
    n62 = global read "JoystickControls.vi" "JoystickControls"() -> (w133:T40)
    n63 = global read "JoystickControls.vi" "JoystickControls"() -> (w126:T40)
    n64 = Unbundle By Name(w157) -> ("H U/D"=w156:dbl)
    n65 = Select(t="ShooterSpeed(rpm)", s=w97, f=0.0) -> (s? t:f=w95:dbl)
    n66 = call "Shooter_Hood_Control_Manual.vi"("Hood_Command"=w156) -> ("ShooterHoodMotorCommand"=w155:dbl)
    n67 = Unbundle By Name(w133) -> ("H L/R"=w134:dbl)
    n68 = Unbundle By Name(w126) -> ("Find Target"=w110:bool)
    n69 = call "ShooterControl.vi"("PIDParams"=w99, "Setpoint (rpm)"=w95, "MotorControlDevRef"=w100) -> ()  [unwired: 7 in]
    n70 = call "Shooter_Hood_Homing.vi"("Controller_Command"=w155, "Home_Position"=w154, "Homing Activated"="HoodHomeActivate", "Reset"="HoodHomeReset", "Hood_Motor_DevRef"=w152, "MotorConfig"=w153) -> ("Homing_State"=w146:T4, "Motor_Output"=w151:dbl, "MotorConfig Out"=w117:T8, "Hood_Motor_DevRefOut"=w118:T29)
    "Hood_Homing_State" <- w146
    n71 = call "Turret_Control_Manual.vi"("Rotate_Command"=w134) -> ("TurretMotorCommand"=w135:dbl)
    n72 = call "Turret_Homing.vi"("Controller_Command"=w135, "Turret_Motor_DefRef"=w105, "Homing Activated"="Turret Homing Activated", "Reset"="TurretHomeReset", "Home_Position"=w136, "MotorConfig"=w103) -> ("Motor_Output"=w139:dbl, "Homing_State"=w140:T4, "Turret_Motor_DefRef Out"=w104:T29, "MotorConfigOut"=w102:T8)  [unwired: 2 in]
    "Turret Homing_State" <- w140
    n73 = Select(t=VisionPipeline."NoZoom" ("pipeline control"), s=w110, f=VisionPipeline."LEDOff" ("pipeline control")) -> (s? t:f=w123:T41)
    n74 = Equal?(x=w146, y=Hood_Homing_State."Homing in Process") -> (x = y?=w144:bool)
    n75 = call "VisionGetTarget.vi"("pipeline control"=w123, "Camera Pitch [deg.]"=w127, "Camera Height[in.]"=w128, "Limelight name"="limelight") -> ("VisionTarget"=w113:T42)  [unwired: 7 in]
    n76 = Equal?(x=w140, y=Hood_Homing_State."Homing in Process") -> (x = y?=w141:bool)
    n77 = call "ShooterHoodPositionControl.vi"("ShooterHoodMotorControlDevRef"=w118, "Activate Auto"="Activate Auto (Shooter Hood)", "MaxDegrees"=w143, "Homing"=w144, "MinDegrees"=w142, "MotorConfig"=w117, "SetPoint(Deg)"="SetPointHood(Deg)", "ManualControl"=w151, "PIDParams"=w119) -> ("Manual?"=→"HoodManual?":bool, "Current Position (Deg)"=→"Hood Current Position (Deg)":dbl)  [unwired: 3 in, 2 out]
    n78 = Unbundle By Name(w113) -> ("Valid"=→"Target Found?":bool)
    n79 = feedback #1() -> (w112:dbl)  [unwired: 1 in]
    n80 = feedback #2(TRUE ("Manual?")) -> (w111:bool)
    n81 = call "TurretSetpointSelect.vi"("TurretManualControlActive"=w111, "ManualSetpointEnable"="DisableLimelight", "CurrentTurretPosition(deg)"=w112, "ManualSetpointActivate"="Activate Auto (Turret)", "VisionTarget"=w113, "Limelight Radius (in)"=w106, "AutoTargetActivate"=w110, "ManualSetpoint(deg)"="SetPointTurret(Deg)") -> ("Setpoint(deg)"=w114:dbl, "ActivateAutoControl"=w115:bool)  [unwired: 2 in]
    n82 = call "TurretAngleControl.vi"("TurretMotorControlDevRef"=w104, "Activate Auto"=w115, "MaxDegrees"=w138, "Homing"=w141, "MinDegrees"=w137, "MotorConfig"=w102, "SetPoint(Deg)"=w114, "ManualControl"=w139, "PIDParams"=w101) -> ("Manual?"=w121:bool, "Current Position (Deg)"=w122:dbl)  [unwired: 5 in]
    "Turret Current Position (Deg)" <- w122
    "TurretManual" <- w121
    n83 = feedback-in #1(w122) -> ()
    n84 = feedback-in #2(w121) -> ()
    n85 = Wait (ms)(milliseconds to wait=u32 20) -> ()  [unwired: 1 out]
  }
